vi "HTML viewer.vi"() -> (1 "URL":string)   [LabVIEW 2011]
panel:
  in  "file path (use dialog)":path=path "C:/Users/mw24/Desktop/default.html"
  in  "html":string="<form name=\"EtFlocSedFi\" action=\"http://designserver.cee.cornell.edu:8080/DesignServer/DesignForm\" method=\"post\">\n\nName: <input type=\"text\" name=\"Name\" autofocus=\"autofocus\" required=\"required\" /><br />\nEmail address: <input type=\"text\" name=\"Email\" required=\"required\" /><br />\nOrganization: <input type=\"text\" name=\"Organization\" /><br />             \nCountry: \n<select id=\"Country\" name=\"Country\">\n<option value=\"US\">United States</option>\n<option value=\"HN\">Honduras</option>\n<option value=\"AF\">Afghanistan</option>\n<option value=\"AX\">Aland Islands</option>\n<option value=\"AL\">Albania</option>\n<option value=\"DZ\">Algeria</option>\n<option value=\"AS\">American Samoa</option>\n<option value=\"AD\">Andorra</option>\n<option value=\"AO\">Angola</option>\n<option value=\"AI\">Anguilla</option>\n<option value=\"AQ\">Antarctica</option>\n<option value=\"AG\">Antigua and Barbuda</option>\n<option value=\"AR\">Argentina</option>\n<option value=\"AM\">Armenia</option>\n<option value=\"AW\">Aruba</option>\n<option value=\"AU\">Australia</option>\n<option value=\"AT\">Austria</option>\n<option value=\"AZ\">Azerbaijan</option>\n<option value=\"BS\">Bahamas</option>\n<option value=\"BH\">Bahrain</option>\n<option value=\"BD\">Bangladesh</option>\n<option value=\"BB\">Barbados</option>\n<option value=\"BY\">Belarus</option>\n<option value=\"BE\">Belgium</option>\n<option value=\"BZ\">Belize</option>\n<option value=\"BJ\">Benin</option>\n<option value=\"BM\">Bermuda</option>\n<option value=\"BT\">Bhutan</option>\n<option value=\"BO\">Bolivia</option>\n<option value=\"BA\">Bosnia and Herzegovina</option>\n<option value=\"BW\">Botswana</option>\n<option value=\"BV\">Bouvet Island</option>\n<option value=\"BR\">Brazil</option>\n<option value=\"IO\">British Indian Ocean Territory</option>\n<option value=\"BN\">Brunei Darussalam</option>\n<option value=\"BG\">Bulgaria</option>\n<option value=\"BF\">Burkina Faso</option>\n<option value=\"BI\">Burundi</option>\n<option value=\"KH\">Cambodia</option>\n<option value=\"CM\">Cameroon</option>\n<option value=\"CA\">Canada</option>\n\n<option value=\"CV\">Cape Verde</option>\n\n<option value=\"KY\">Cayman Islands</option>\n\n<option value=\"CF\">Central African Republic</option>\n\n<option value=\"TD\">Chad</option>\n\n<option value=\"CL\">Chile</option>\n\n<option value=\"CN\">China</option>\n\n<option value=\"CX\">Christmas Island</option>\n\n<option value=\"CC\">Cocos (Keeling) Islands</option>\n\n<option value=\"CO\">Colombia</option>\n\n<option value=\"KM\">Comoros</option>\n\n<option value=\"CG\">Congo</option>\n\n<option value=\"CD\">Congo, The Democratic Republic of The</option>\n\n<option value=\"CK\">Cook Islands</option>\n\n<option value=\"CR\">Costa Rica</option>\n\n<option value=\"CI\">Cote D'ivoire</option>\n\n<option value=\"HR\">Croatia</option>\n\n<option value=\"CU\">Cuba</option>\n\n<option value=\"CY\">Cyprus</option>\n\n<option value=\"CZ\">Czech Republic</option>\n\n<option value=\"DK\">Denmark</option>\n\n<option value=\"DJ\">Djibouti</option>\n\n<option value=\"DM\">Dominica</option>\n\n<option value=\"DO\">Dominican Republic</option>\n\n<option value=\"EC\">Ecuador</option>\n\n<option value=\"EG\">Egypt</option>\n\n<option value=\"SV\">El Salvador</option>\n\n<option value=\"GQ\">Equatorial Guinea</option>\n\n<option value=\"ER\">Eritrea</option>\n\n<option value=\"EE\">Estonia</option>\n\n<option value=\"ET\">Ethiopia</option>\n\n<option value=\"FK\">Falkland Islands (Malvinas)</option>\n\n<option value=\"FO\">Faroe Islands</option>\n\n<option value=\"FJ\">Fiji</option>\n\n<option value=\"FI\">Finland</option>\n\n<option value=\"FR\">France</option>\n\n<option value=\"GF\">French Guiana</option>\n\n<option value=\"PF\">French Polynesia</option>\n\n<option value=\"TF\">French Southern Territories</option>\n\n<option value=\"GA\">Gabon</option>\n\n<option value=\"GM\">Gambia</option>\n\n<option value=\"GE\">Georgia</option>\n\n<option value=\"DE\">Germany</option>\n\n<option value=\"GH\">Ghana</option>\n\n<option value=\"GI\">Gibraltar</option>\n\n<option value=\"GR\">Greece</option>\n\n<option value=\"GL\">Greenland</option>\n\n<option value=\"GD\">Grenada</option>\n\n<option value=\"GP\">Guadeloupe</option>\n\n<option value=\"GU\">Guam</option>\n\n<option value=\"GT\">Guatemala</option>\n\n<option value=\"GG\">Guernsey</option>\n\n<option value=\"GN\">Guinea</option>\n\n<option value=\"GW\">Guinea-bissau</option>\n\n<option value=\"GY\">Guyana</option>\n\n<option value=\"HT\">Haiti</option>\n\n<option value=\"HM\">Heard Island and Mcdonald Islands</option>\n\n<option value=\"VA\">Holy See (Vatican City State)</option>\n\n<option value=\"HK\">Hong Kong</option>\n\n<option value=\"HU\">Hungary</option>\n\n<option value=\"IS\">Iceland</option>\n\n<option value=\"IN\">India</option>\n\n<option value=\"ID\">Indonesia</option>\n\n<option value=\"IR\">Iran, Islamic Republic of</option>\n\n<option value=\"IQ\">Iraq</option>\n\n<option value=\"IE\">Ireland</option>\n\n<option value=\"IM\">Isle of Man</option>\n\n<option value=\"IL\">Israel</option>\n\n<option value=\"IT\">Italy</option>\n\n<option value=\"JM\">Jamaica</option>\n\n<option value=\"JP\">Japan</option>\n\n<option value=\"JE\">Jersey</option>\n\n<option value=\"JO\">Jordan</option>\n\n<option value=\"KZ\">Kazakhstan</option>\n\n<option value=\"KE\">Kenya</option>\n\n<option value=\"KI\">Kiribati</option>\n\n<option value=\"KP\">Korea, Democratic People's Republic of</option>\n\n<option value=\"KR\">Korea, Republic of</option>\n\n<option value=\"KW\">Kuwait</option>\n\n<option value=\"KG\">Kyrgyzstan</option>\n\n<option value=\"LA\">Lao People's Democratic Republic</option>\n\n<option value=\"LV\">Latvia</option>\n\n<option value=\"LB\">Lebanon</option>\n\n<option value=\"LS\">Lesotho</option>\n\n<option value=\"LR\">Liberia</option>\n\n<option value=\"LY\">Libyan Arab Jamahiriya</option>\n\n<option value=\"LI\">Liechtenstein</option>\n\n<option value=\"LT\">Lithuania</option>\n\n<option value=\"LU\">Luxembourg</option>\n\n<option value=\"MO\">Macao</option>\n\n<option value=\"MK\">Macedonia, The Former Yugoslav Republic of</option>\n\n<option value=\"MG\">Madagascar</option>\n\n<option value=\"MW\">Malawi</option>\n\n<option value=\"MY\">Malaysia</option>\n\n<option value=\"MV\">Maldives</option>\n\n<option value=\"ML\">Mali</option>\n\n<option value=\"MT\">Malta</option>\n\n<option value=\"MH\">Marshall Islands</option>\n\n<option value=\"MQ\">Martinique</option>\n\n<option value=\"MR\">Mauritania</option>\n\n<option value=\"MU\">Mauritius</option>\n\n<option value=\"YT\">Mayotte</option>\n\n<option value=\"MX\">Mexico</option>\n\n<option value=\"FM\">Micronesia, Federated States of</option>\n\n<option value=\"MD\">Moldova, Republic of</option>\n\n<option value=\"MC\">Monaco</option>\n\n<option value=\"MN\">Mongolia</option>\n\n<option value=\"ME\">Montenegro</option>\n\n<option value=\"MS\">Montserrat</option>\n\n<option value=\"MA\">Morocco</option>\n\n<option value=\"MZ\">Mozambique</option>\n\n<option value=\"MM\">Myanmar</option>\n\n<option value=\"NA\">Namibia</option>\n\n<option value=\"NR\">Nauru</option>\n\n<option value=\"NP\">Nepal</option>\n\n<option value=\"NL\">Netherlands</option>\n\n<option value=\"AN\">Netherlands Antilles</option>\n\n<option value=\"NC\">New Caledonia</option>\n\n<option value=\"NZ\">New Zealand</option>\n\n<option value=\"NI\">Nicaragua</option>\n\n<option value=\"NE\">Niger</option>\n\n<option value=\"NG\">Nigeria</option>\n\n<option value=\"NU\">Niue</option>\n\n<option value=\"NF\">Norfolk Island</option>\n\n<option value=\"MP\">Northern Mariana Islands</option>\n\n<option value=\"NO\">Norway</option>\n\n<option value=\"OM\">Oman</option>\n\n<option value=\"PK\">Pakistan</option>\n\n<option value=\"PW\">Palau</option>\n\n<option value=\"PS\">Palestinian Territory, Occupied</option>\n\n<option value=\"PA\">Panama</option>\n\n<option value=\"PG\">Papua New Guinea</option>\n\n<option value=\"PY\">Paraguay</option>\n\n<option value=\"PE\">Peru</option>\n\n<option value=\"PH\">Philippines</option>\n\n<option value=\"PN\">Pitcairn</option>\n\n<option value=\"PL\">Poland</option>\n\n<option value=\"PT\">Portugal</option>\n\n<option value=\"PR\">Puerto Rico</option>\n\n<option value=\"QA\">Qatar</option>\n\n<option value=\"RE\">Reunion</option>\n\n<option value=\"RO\">Romania</option>\n\n<option value=\"RU\">Russian Federation</option>\n\n<option value=\"RW\">Rwanda</option>\n\n<option value=\"SH\">Saint Helena</option>\n\n<option value=\"KN\">Saint Kitts and Nevis</option>\n\n<option value=\"LC\">Saint Lucia</option>\n\n<option value=\"PM\">Saint Pierre and Miquelon</option>\n\n<option value=\"VC\">Saint Vincent and The Grenadines</option>\n\n<option value=\"WS\">Samoa</option>\n\n<option value=\"SM\">San Marino</option>\n\n<option value=\"ST\">Sao Tome and Principe</option>\n\n<option value=\"SA\">Saudi Arabia</option>\n\n<option value=\"SN\">Senegal</option>\n\n<option value=\"RS\">Serbia</option>\n\n<option value=\"SC\">Seychelles</option>\n\n<option value=\"SL\">Sierra Leone</option>\n\n<option value=\"SG\">Singapore</option>\n\n<option value=\"SK\">Slovakia</option>\n\n<option value=\"SI\">Slovenia</option>\n\n<option value=\"SB\">Solomon Islands</option>\n\n<option value=\"SO\">Somalia</option>\n\n<option value=\"ZA\">South Africa</option>\n\n<option value=\"GS\">South Georgia and The South Sandwich Islands</option>\n\n<option value=\"ES\">Spain</option>\n\n<option value=\"LK\">Sri Lanka</option>\n\n<option value=\"SD\">Sudan</option>\n\n<option value=\"SR\">Suriname</option>\n\n<option value=\"SJ\">Svalbard and Jan Mayen</option>\n\n<option value=\"SZ\">Swaziland</option>\n\n<option value=\"SE\">Sweden</option>\n\n<option value=\"CH\">Switzerland</option>\n\n<option value=\"SY\">Syrian Arab Republic</option>\n\n<option value=\"TW\">Taiwan, Province of China</option>\n\n<option value=\"TJ\">Tajikistan</option>\n\n<option value=\"TZ\">Tanzania, United Republic of</option>\n\n<option value=\"TH\">Thailand</option>\n\n<option value=\"TL\">Timor-leste</option>\n\n<option value=\"TG\">Togo</option>\n\n<option value=\"TK\">Tokelau</option>\n\n<option value=\"TO\">Tonga</option>\n\n<option value=\"TT\">Trinidad and Tobago</option>\n\n<option value=\"TN\">Tunisia</option>\n\n<option value=\"TR\">Turkey</option>\n\n<option value=\"TM\">Turkmenistan</option>\n\n<option value=\"TC\">Turks and Caicos Islands</option>\n\n<option value=\"TV\">Tuvalu</option>\n\n<option value=\"UG\">Uganda</option>\n\n<option value=\"UA\">Ukraine</option>\n\n<option value=\"AE\">United Arab Emirates</option>\n\n<option value=\"GB\">United Kingdom</option>\n\n<option value=\"UM\">United States Minor Outlying Islands</option>\n\n<option value=\"UY\">Uruguay</option>\n\n<option value=\"UZ\">Uzbekistan</option>\n\n<option value=\"VU\">Vanuatu</option>\n\n<option value=\"VE\">Venezuela</option>\n\n<option value=\"VN\">Viet Nam</option>\n\n<option value=\"VG\">Virgin Islands, British</option>\n\n<option value=\"VI\">Virgin Islands, U.S.</option>\n\n<option value=\"WF\">Wallis and Futuna</option>\n\n<option value=\"EH\">Western Sahara</option>\n\n<option value=\"YE\">Yemen</option>\n\n<option value=\"ZM\">Zambia</option>\n\n<option value=\"ZW\">Zimbabwe</option>\n\n</select><br />\n\n\t\t\t \tProject Title: <input type=\"text\" name=\"ProjectTitle\" /><br />    \n\nProject City: <input type=\"text\" name=\"ProjectCity\" /><br />\n\nProject State: <input type=\"text\" name=\"ProjectState\" /><br />    \n\nProject Notes: <input type=\"text\" name=\"ProjectNotes\" /><br />  <br />\n\n\t\t\t \t<br />\tFlow Rate (L/s): <input type=\"number\" name=\"Q.Plant[L/s]\" min=\"3\" max=\"90\" step=\".5\" value=\"18\" required=\"required\" /> \n\n\t\t\t \t\n\n                \t\t\t<input type=\"submit\" value=\"Get a Design\" />\n\n            \t\t\t</form>"
  in  "OK Button":bool
  in  "WebBrowser":refnum<k7>(container)
  # "file:///C:/Users/mw24/Desktop/default.html"
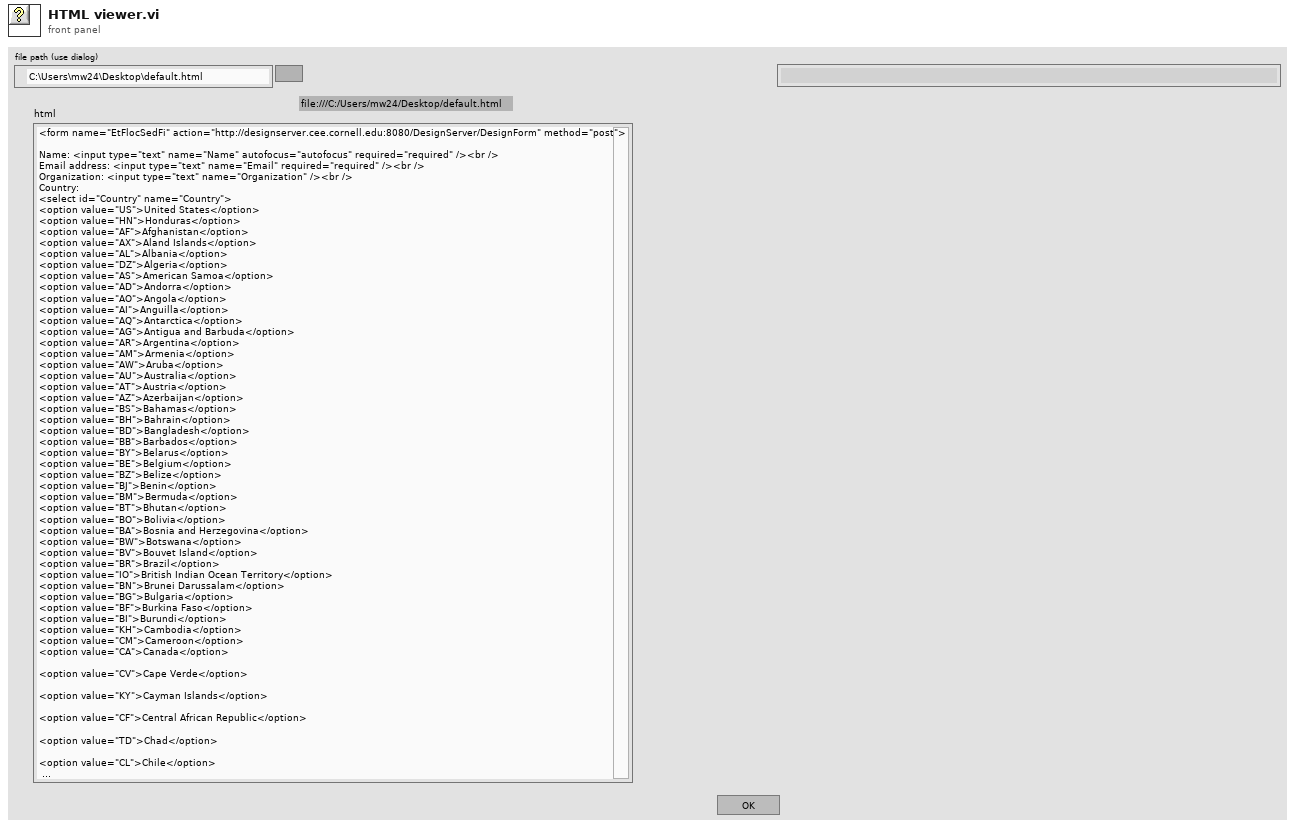
[diagram p1: front panel]
types:
  T1 = enum16{"open", "replace", "create", "open or create", "replace or create", "replace or create with confirmation"}
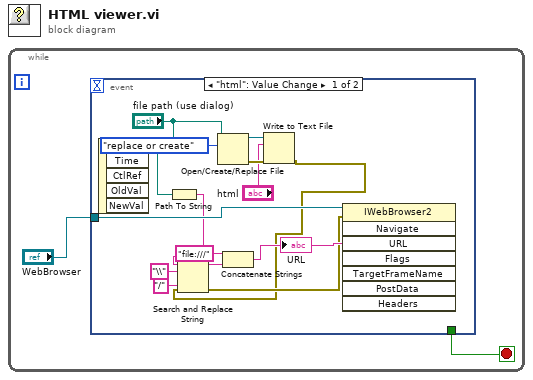
[diagram p0: block diagram]
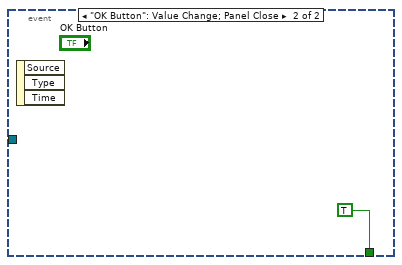
[diagram p2: hidden frame]
diagram:
  n1 = while {
    stop <- w2 stop-if-true
    n2 = event shown="[0] \"html\": Value Change" {
      selector: _ -> [_ _]
      dyn-events: _ -> [_ _]
      timeout: _ -> [_ _]
      tunnel: [_ TRUE] -> w2
      tunnel: "WebBrowser" -> [w16 _]
      event "html": Value Change {
        n3 = event-data() -> ()  [unwired: 1 in, 5 out]
        n4 = Path To String(path="file path (use dialog)") -> (string=w10:string)
        n5 = Open/Create/Replace File(file path (use dialog)="file path (use dialog)", operation (0:open)=T1."replace or create") -> (refnum out=w14:refnum<file>, error out=w15:errorcluster)  [unwired: 4 in, 1 out]
        n6 = Write to Text File(file (use dialog)=w14, text="html", error in=w15) -> (error out=w3:errorcluster)  [unwired: 1 in, 2 out]
        n7 = Search and Replace String(input string=w10, search string="\\", replace string="/" ("replace string (\"\")"), error in=w3) -> (result string=w7:string, error out=w4:errorcluster)  [unwired: 4 in, 2 out]
        n8 = Concatenate Strings("file:///" ("string"), w7) -> (w5:string)
        "URL" <- w5
        n9 = invoke class="IWebBrowser2" method="Navigate"(reference=w16, error in=w4, "URL"=w5) -> ()  [unwired: 5 in, 8 out]
      }
      event "OK Button": Value Change; Panel Close {
        n10 = event-data() -> ()  [unwired: 1 in, 3 out]
      }
    }
  }
